vi "VTI_Merge_Cluster.vi"(1 "VTI Control":T1, 2 "VTI Status":T3={"Temperatur (K)"=70.6986, "Heater (%)"=0.0017142857142857142, "NV (%)"=0.0, "Heater Manual"=TRUE, "NV Manual"=TRUE, "Pressure"=1.0208606, "Valid?"=FALSE, "Heater (%) Display"=0.0, "NV (%) Display"=0.0, "Sample 2"=70.6986, "Sample 3"=70.6986, "Auto PID"=TRUE, "Sweep-Status"=TRUE, "Setpoint-Sweep"=70.6986} {"Heater (%)" scale=0.0..100.0; "NV (%)" scale=0.0..100.0}) -> (0 "VTI":T2={"Temperatur (K)"=0.0, "Setpoint (K)"=0.0, "Rate (K/min)"=3.4572, "Heater (%)"=0.0, "NV (%)"=0.0, "Heater Manual"=FALSE, "NV Manual"=FALSE, "Go to Set"=FALSE, "Pressure"=0.0, "Heater SP"=0.0, "Valid?"=FALSE, "Set Heater SP"=FALSE, "Set NV SP"=FALSE, "Heater (%) Display"=3.4572, "NV (%) Display"=3.4572, "NV Setpoint"=0.0, "Change Heater Status"=FALSE, "Change NV Status"=FALSE, "Sample 3"=0.0, "Sample 2"=0.0, "Sweep-State"=FALSE, "Set Auto PID"=FALSE, "Auto PID"=FALSE, "Stopp"=FALSE, "Setpoint-Sweep"=0.0} {"NV (%) Display" format="%4_5f"; "Heater (%) Display" format="%4_5f"; "Pressure" format="%#4_5f"; "NV (%)" scale=0.0..100.0; "Heater (%)" scale=0.0..100.0; "Rate (K/min)" format="%#4_5f"; "Setpoint (K)" format="%6_5f"})   [LabVIEW 2019]
uses:
  S16/VTI-status.ctl
  S16/VTI-cluster.ctl
  S16/VTI-control.ctl
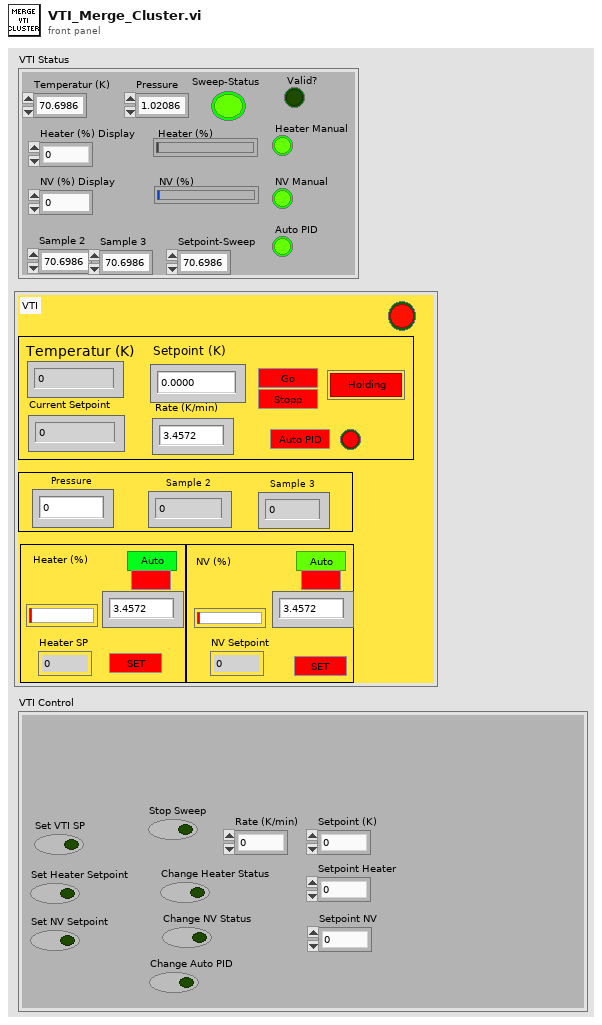
[diagram p1: front panel]
types:
  T1 = typedef "VTI-control.ctl" = cluster{"Set VTI SP":bool, "Change NV Status":bool, "Set NV Setpoint":bool, "Change Heater Status":bool, "Set Heater Setpoint":bool, "Setpoint (K)":dbl, "Rate (K/min)":dbl, "Setpoint Heater":dbl, "Setpoint NV":dbl, "Change Auto PID":bool, "Stop Sweep":bool}
  T2 = typedef "VTI-cluster.ctl" = cluster{"Temperatur (K)":dbl, "Setpoint (K)":dbl, "Rate (K/min)":dbl, "Heater (%)":dbl, "NV (%)":dbl, "Heater Manual":bool, "NV Manual":bool, "Go to Set":bool, "Pressure":dbl, "Heater SP":dbl, "Valid?":bool, "Set Heater SP":bool, "Set NV SP":bool, "Heater (%) Display":dbl, "NV (%) Display":dbl, "NV Setpoint":dbl, "Change Heater Status":bool, "Change NV Status":bool, "Sample 3":dbl, "Sample 2":dbl, "Sweep-State":bool, "Set Auto PID":bool, "Auto PID":bool, "Stopp":bool, "Setpoint-Sweep":dbl}
  T3 = typedef "VTI-status.ctl" = cluster{"Temperatur (K)":dbl, "Heater (%)":dbl, "NV (%)":dbl, "Heater Manual":bool, "NV Manual":bool, "Pressure":dbl, "Valid?":bool, "Heater (%) Display":dbl, "NV (%) Display":dbl, "Sample 2":dbl, "Sample 3":dbl, "Auto PID":bool, "Sweep-Status":bool, "Setpoint-Sweep":dbl}
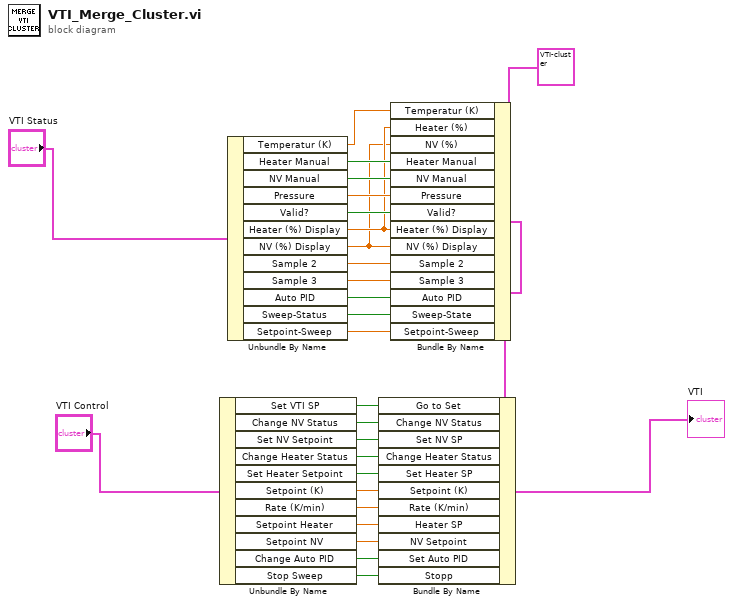
[diagram p0: block diagram]
diagram:
  n1 = Unbundle By Name("VTI Control") -> ("Set VTI SP"=w28:bool, "Change NV Status"=w27:bool, "Set NV Setpoint"=w26:bool, "Change Heater Status"=w20:bool, "Set Heater Setpoint"=w21:bool, "Setpoint (K)"=w22:dbl, "Rate (K/min)"=w23:dbl, "Setpoint Heater"=w24:dbl, "Setpoint NV"=w25:dbl, "Change Auto PID"=w7:bool, "Stop Sweep"=w5:bool)
  n2 = Unbundle By Name("VTI Status") -> ("Temperatur (K)"=w3:dbl, "Heater Manual"=w19:bool, "NV Manual"=w18:bool, "Pressure"=w17:dbl, "Valid?"=w16:bool, "Heater (%) Display"=w2:dbl, "NV (%) Display"=w1:dbl, "Sample 2"=w10:dbl, "Sample 3"=w9:dbl, "Auto PID"=w8:bool, "Sweep-Status"=w6:bool, "Setpoint-Sweep"=w4:dbl)
  n3 = Bundle By Name(cluster=T2 {"Temperatur (K)"=0.0, "Setpoint (K)"=0.0, "Rate (K/min)"=0.0, "Heater (%)"=0.0, "NV (%)"=0.0, "Heater Manual"=FALSE, "NV Manual"=FALSE, "Go to Set"=FALSE, "Pressure"=0.0, "Heater SP"=0.0, "Valid?"=FALSE, "Set Heater SP"=FALSE, "Set NV SP"=FALSE, "Heater (%) Display"=0.0, "NV (%) Display"=0.0, "NV Setpoint"=0.0, "Change Heater Status"=FALSE, "Change NV Status"=FALSE, "Sample 3"=0.0, "Sample 2"=0.0, "Sweep-State"=FALSE, "Set Auto PID"=FALSE, "Auto PID"=FALSE, "Stopp"=FALSE, "Setpoint-Sweep"=0.0} ("VTI 2"), "Temperatur (K)"=w3, "Heater (%)"=w2, "NV (%)"=w1, "Heater Manual"=w19, "NV Manual"=w18, "Pressure"=w17, "Valid?"=w16, "Heater (%) Display"=w2, "NV (%) Display"=w1, "Sample 2"=w10, "Sample 3"=w9, "Auto PID"=w8, "Sweep-State"=w6, "Setpoint-Sweep"=w4) -> (w13:T2)
  n4 = Bundle By Name(cluster=w13, "Go to Set"=w28, "Change NV Status"=w27, "Set NV SP"=w26, "Change Heater Status"=w20, "Set Heater SP"=w21, "Setpoint (K)"=w22, "Rate (K/min)"=w23, "Heater SP"=w24, "NV Setpoint"=w25, "Set Auto PID"=w7, "Stopp"=w5) -> (→"VTI":T2)
